vi "test Controller.vi"(8 "error in":errorcluster) -> ()   [LabVIEW 2020]
doc: "This VI executes continuously carrying out the current operation and responding to updates or new operations. It will often contain the timing or control code that is difficult to place directly in TeleOp. This VI generally opens all sensors and motors and isolates the rest of the robot code from knowing how the operations are carried out."
uses:
  <vilib>/Rock Robotics/Network Tables/NT Write Boolean.vi
  test Setpoints.ctl
  test Operations.ctl
  <vilib>/Rock Robotics/WPI/Framework/Completion Status.ctl
panel:
  in  "Interactive Values":T1
  out "Current\nCmd":string
  in  "Buttons":cluster{"Execute Cmd":bool, "Abort Cmd":bool}
  out "Command Timing":cluster{"Start Time (ms)":u32, "Iterations":i32}
  out "Status":T3
  # "Tip: It may be helpful to observe inputs and sensor values.\nYou may also want to display tuning or debugging controls."
  # "Interactive Command: You may fill in the settings for a command\nand schedule it with the Execute button. You can observe and abort\nany command while fine tuning the code for the controller."
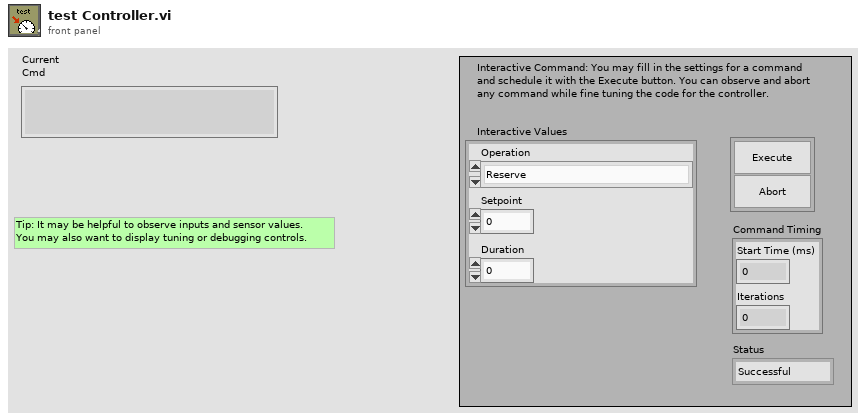
[diagram p1: front panel]
types:
  T1 = typedef "test Setpoints.ctl" = cluster{"Operation":T2, "Setpoint":dbl, "Duration":dbl}
  T2 = typedef "test Operations.ctl" = enum16{"Reserve", "Read Current", "Immediate", "For Time", "Stop"}
  T3 = typedef "Completion Status.ctl" = enum16{"Successful", "Aborted", "Incomplete"}
  T4 = typedef "Command Status Info.ctl" = cluster{"Name":string, "Status":T3, "notifier out":T5}
  T5 = typedef "Completion Notifier.ctl" = refnum<notifier>
  T6 = cluster{"Current Command":T1, "Command Timing":cluster{"Start Time (ms)":u32, "Iterations":i32}, "Command Arguments":cluster{"Command Info":T4, "Description":string, "Default Command":T1, "queue out":refnum<queue>, "Subsystem Name":string}}
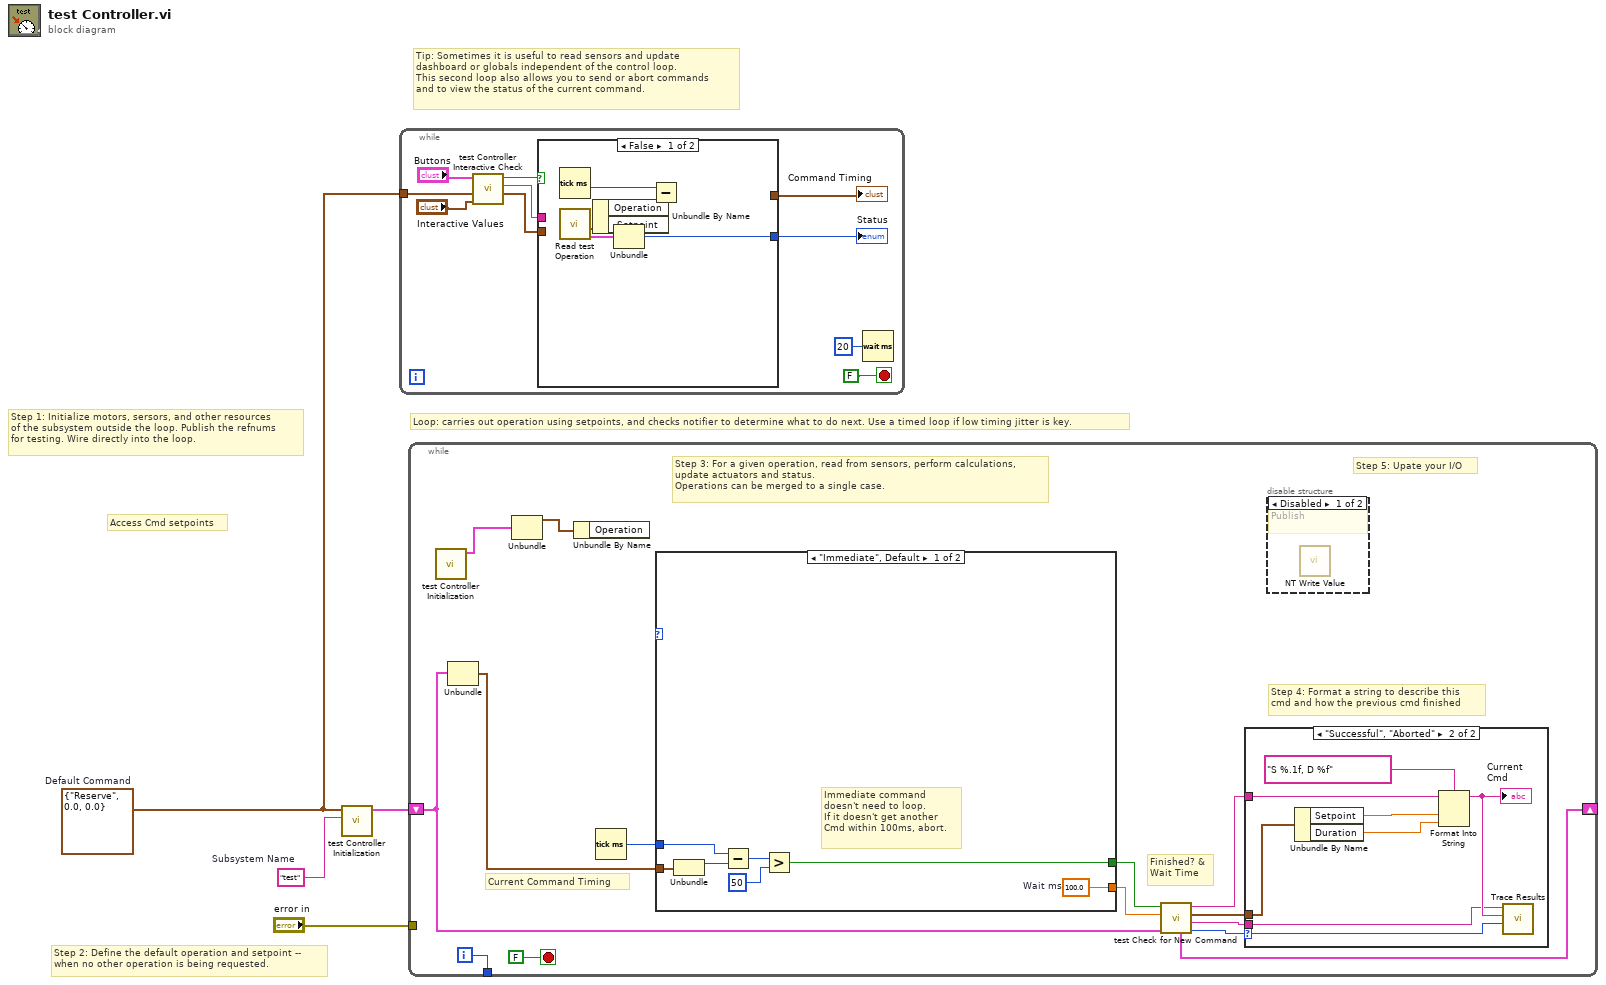
[diagram p0: block diagram]
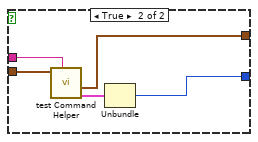
[diagram p2: hidden frame]
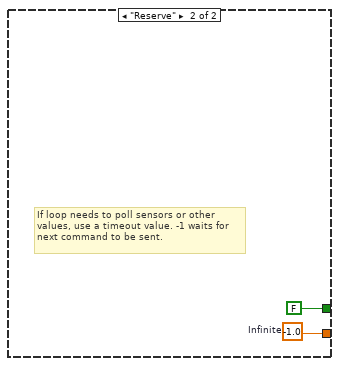
[diagram p5: hidden frame]
diagram:
  w1 = T1 {"Operation"=enum."Reserve", "Setpoint"=0.0, "Duration"=0.0}  # Default Command
  w2 = "test"  # Subsystem Name
  # "Access Cmd setpoints"
  # "Tip: Sometimes it is useful to read sensors and update\ndashboard or globals independent of the control loop.\nThis second loop also allows you to send or abort commands\nand to view the status of the current command."
  # "Step 2: Define the default operation and setpoint --\nwhen no other operation is being requested."
  # "Step 1: Initialize motors, sersors, and other resources\nof the subsystem outside the loop. Publish the refnums\nfor testing. Wire directly into the loop."
  # "Loop: carries out operation using setpoints, and checks notifier to determine what to do next. Use a timed loop if low timing jitter is key."
  n1 = call "test Controller Initialization.vi"("Subsystem Name"=w2, "Default Command"=w1) -> ("Current Command"=w3:T6)  [unwired: 9 in]
  n2 = while {
    tunnel: w1 -> [w11]
    stop <- FALSE stop-if-true
    n3 = call "test Controller Interactive Check.vi"("Interactive Command in"="Interactive Values", "Default Command"=w11, "Buttons"="Buttons") -> ("Interactive Command out"=w8:T1, "Trace String"=w9:string, "Schedule"=w10:bool)  [unwired: 6 in]
    n4 = case shown="False" w10 {
      tunnel: [w18 w23] -> w7
      tunnel: w8 -> [_ w21]
      tunnel: [_ w19] -> w6
      tunnel: w9 -> [_ w22]
      frame False {
        n5 = Tick Count (ms)() -> (millisecond timer value=w17:u32)
        n6 = call "Read test Operation.vi"() -> ("Command Info"=w16:T4, "SubSystem Data"=w15:T1)  [unwired: 9 in, 1 out]
        n7 = Unbundle By Name(w15) -> ()  [unwired: 2 out]
        n8 = Unbundle(w16) -> ("Status"=w18:T3)  [unwired: 2 out]
        n9 = Subtract(x=w17) -> ()  [unwired: 1 in, 1 out]
      }
      frame True {
        n10 = call "test Command Helper.vi"("Description"=w22, "SubSystem Data"=w21) -> ("Command Info Out"=w20:T4, "Command Timing"=w19:cluster{"Start Time (ms)":u32, "Iterations":i32})  [unwired: 7 in, 1 out]
        n11 = Unbundle(w20) -> ("Status"=w23:T3)  [unwired: 2 out]
      }
    }
    "Status" <- w7
    "Command Timing" <- w6
    n12 = Wait (ms)(milliseconds to wait=u32 20) -> ()  [unwired: 1 out]
  }
  n13 = while {
    shift-right: [w34] -> _
    shift-left: w3 -> [w25]
    tunnel: [w37] -> _
    tunnel: "error in" -> [_]
    i -> [w37]
    stop <- FALSE stop-if-true
    # "Step 5: Upate your I/O"
    # "Step 4: Format a string to describe this\ncmd and how the previous cmd finished"
    # "Current Command Timing"
    # "Finished? &\nWait Time"
    # "Step 3: For a given operation, read from sensors, perform calculations,\nupdate actuators and status.\nOperations can be merged to a single case."
    n14 = call "test Controller Initialization.vi"() -> ("Current Command"=w27:T6)  [unwired: 11 in]
    n15 = Unbundle(w25) -> ("Command Timing"=w24:cluster{"Start Time (ms)":u32, "Iterations":i32})  [unwired: 2 out]
    n16 = Unbundle(w27) -> ("Current Command"=w26:T1)  [unwired: 2 out]
    n17 = Unbundle By Name(w26) -> ()  [unwired: 1 out]
    n18 = Tick Count (ms)() -> (millisecond timer value=w35:u32)
    n19 = case shown="\"Immediate\", Default" w36 {
      tunnel: [w53 w55] -> w32
      tunnel: [w47 FALSE ("ignore previous (F)")] -> w33
      tunnel: w24 -> [w49 _]
      tunnel: w35 -> [w48 _]
      frame "Immediate", Default {
        w53 = 100.0  # Wait ms
        # "Immediate command\ndoesn't need to loop.\nIf it doesn't get another\nCmd within 100ms, abort."
        n20 = Unbundle(w49) -> ("Start Time (ms)"=w52:u32)  [unwired: 1 out]
        n21 = Subtract(x=w48, y=w52) -> (x-y=w51:u32)
        n22 = Greater?(x=w51, y=u8 50 ("Left Motor")) -> (0:w47:bool)
      }
      frame "Reserve" {
        w55 = -1.0  # Infinite
        # "If loop needs to poll sensors or other\nvalues, use a timeout value. -1 waits for\nnext command to be sent."
      }
    }
    n23 = call "test Check for New Command.vi"("Current Command"=w25, "Wait time (ms)"=w32, "Finished?"=w33) -> ("Completion"=w28:T3, "Subsystem Name"=w29:string, "Current Command"=w30:T1, "Initial Trace String"=w31:string, "NextCommand"=w34:T6)  [unwired: 4 in]
    n24 = case shown="\"Successful\", \"Aborted\"" w28 {
      selector: w28 -> [_ w46]
      tunnel: w31 -> [_ w42]
      tunnel: w30 -> [_ w43]
      tunnel: w29 -> [_ w39]
      frame "Incomplete", Default {
        # "Continuing current command"
      }
      frame "Successful", "Aborted" {
        # "Report and setup for next command"
        n25 = Unbundle By Name(w43) -> ("Setpoint"=w45:dbl, "Duration"=w40:dbl)
        n26 = Format Into String(format string="S %.1f, D %f", initial string=w42, w45, w40) -> (resulting string=w41:string)  [unwired: 1 in, 1 out]
        "Current\nCmd" <- w41
        n27 = call <vilib>:"Trace Results.vi"("Status of previous command"=w46, "Description"=w41, "Subsystem"=w39) -> ()  [unwired: 9 in]
      }
    }
    n28 = disable-structure shown="Disabled" {
      frame Disabled {
        # "Publish"
        n29 = call-poly <vilib>:"NT Write Value.vi"() -> ()  [unwired: 11 in, 1 out]
      }
      frame Enabled {
      }
    }
  }
